vi "MainGui.Buttons.Show.vi"(0 "Show (F)":bool, 1 "Btns":refnum<vi>[](array[refnum])) -> ()   [LabVIEW 2016]
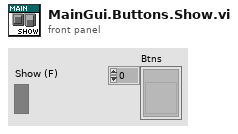
[diagram p1: front panel]
types:
  T1 = enum8{"Enabled", "Disabled", "Disabled and Grayed Out"}
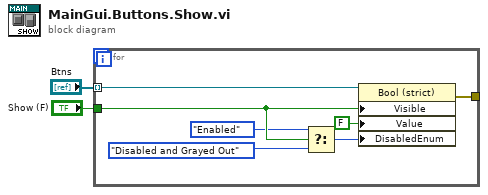
[diagram p0: block diagram]
diagram:
  n1 = for {
    tunnel: "Btns" -> [w9] mode=indexing
    tunnel: [w8] -> _
    tunnel: "Show (F)" -> [w7]
    n2 = Select(t=T1."Enabled" ("Disabled"), s=w7, f=T1."Disabled and Grayed Out" ("Disabled")) -> (s? t:f=w5:T1)
    n3 = property class="Bool (strict)"(reference=w9, "Visible"=w7, "Value"=FALSE, "DisabledEnum"=w5) -> (error out=w8:errorcluster)  [unwired: 1 in, 1 out]
  }
